vi "LFA_AcquireAltSPEMethod.vi"(8 "error in (no error)":errorcluster, 10 "Delete File?":bool, 11 "LightField Automation in":refnum<class "LightField Automation.lvclass">) -> (0 "error out":errorcluster, 2 "Data":T1(array[cluster]), 3 "LightField Automation out":refnum<class "LightField Automation.lvclass">)   [LabVIEW 2020, in "LightField Automation.lvclass"]
uses:
  LightField Automation.lvclass
  LightField Automation.lvclass/LightField Automation.ctl
  C:/Program Files/Princeton Instruments/LightField/AddInViews/PrincetonInstruments.LightFieldViewV3.dll
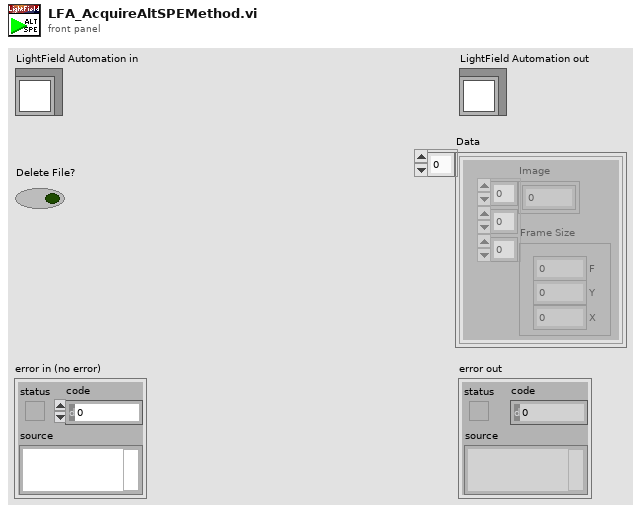
[diagram p1: front panel]
types:
  T1 = cluster{"Image":dbl[][][], "Frame Size":cluster{"F":i32, "Y":i32, "X":i32}}[]
  T2 = cluster{"ROI Height":i32[], "ROI Width":i32[], "ROI Stride":i32[], "ROI Size":i64[]}
  T3 = cluster{"Pixel Format":string, "Number of Frames":i32, "Frame Size":i32, "Frame Stride":i64}
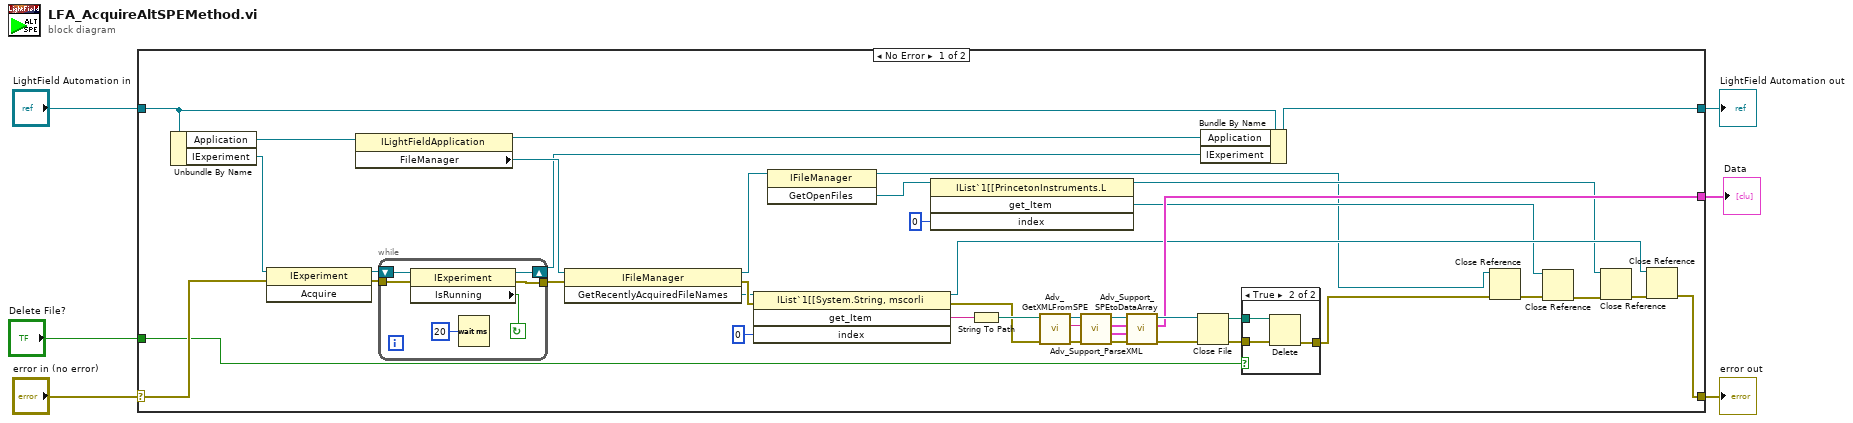
[diagram p0: block diagram]
diagram:
  n1 = case shown="No Error" "error in (no error)" {
    selector: "error in (no error)" -> [w48 w60]
    tunnel: [w20 w60] -> w5
    tunnel: [w26 w59] -> w3
    tunnel: "LightField Automation in" -> [w27 w59]
    tunnel: [w25 _] -> w2
    tunnel: "Delete File?" -> [w22 _]
    frame No Error {
      n2 = Unbundle By Name(w27) -> ("Application"=w44:refnum<k24>, "IExperiment"=w45:refnum<k24>)
      n3 = invoke class="IExperiment" method="Acquire"(reference=w45, error in=w48) -> (reference out=w46:refnum<k24>, error out=w47:errorcluster)  [unwired: 1 in, 1 out]
      n4 = property class="ILightFieldApplication"(reference=w44) -> (reference out=w16:refnum<k24>, "FileManager"=w43:refnum<k24>)  [unwired: 1 in, 1 out]
      n5 = while {
        tunnel: w47 -> [w56]
        tunnel: [w55] -> w42
        shift-right: [w53] -> w21
        shift-left: w46 -> [w54]
        stop <- w58 continue-if-true
        n6 = property class="IExperiment"(reference=w54, error in=w56) -> (reference out=w53:refnum<k24>, error out=w55:errorcluster, "IsRunning"=w58:bool)
        n7 = Wait (ms)(milliseconds to wait=u32 20) -> ()  [unwired: 1 out]
      }
      n8 = invoke class="IFileManager" method="GetRecentlyAcquiredFileNames"(reference=w43, error in=w42) -> (reference out=w15:refnum<k24>, error out=w41:errorcluster, "GetRecentlyAcquiredFileNames"=w19:refnum<k24>)  [unwired: 1 in]
      n9 = invoke class="IList`1[[System.String, mscorli" method="get_Item"(reference=w19, error in=w41, "index"=0) -> (reference out=w17:refnum<k24>, error out=w37:errorcluster, "get_Item"=w39:string)  [unwired: 1 in, 1 out]
      n10 = invoke class="IFileManager" method="GetOpenFiles"(reference=w15) -> (reference out=w7:refnum<k24>, "GetOpenFiles"=w14:refnum<k24>)  [unwired: 2 in, 1 out]
      n11 = invoke class="IList`1[[PrincetonInstruments.L" method="get_Item"(reference=w14, "index"=0) -> (reference out=w12:refnum<k24>, "get_Item"=w9:refnum<k24>)  [unwired: 2 in, 2 out]
      n12 = String To Path(string=w39) -> (path=w38:path)
      n13 = call "Adv_GetXMLFromSPE.vi"("error in (no error)"=w37, "Path In"=w38) -> ("error out"=w34:errorcluster, "XML"=w35:string, "SPE Refnum"=w36:refnum<file>)  [unwired: 7 in]
      n14 = call "Adv_Support_ParseXML.vi"("error in (no error)"=w34, "XML"=w35, "SPE Refnum"=w36) -> ("error out"=w30:errorcluster, "ROI Info"=w31:T2, "Frame Info"=w32:T3, "SPE Refnum"=w33:refnum<file>)  [unwired: 5 in]
      n15 = call "Adv_Support_SPEtoDataArray.vi"("error in (no error)"=w30, "ROI Info"=w31, "Frame Info"=w32, "SPE Refnum"=w33) -> ("error out"=w29:errorcluster, "Data"=w25:T1, "SPE Refnum 2"=w28:refnum<file>)  [unwired: 5 in]
      n16 = Close File(refnum=w28, error in=w29) -> (path=w23:path, error out=w24:errorcluster)
      n17 = Bundle By Name(cluster=w27, "Application"=w16, "IExperiment"=w21) -> (w26:refnum<class "LightField Automation.lvclass">)
      n18 = case shown="True" w22 {
        tunnel: w24 -> [w49 w52]
        tunnel: w23 -> [_ w51]
        tunnel: [w49 w50] -> w8
        frame False {
        }
        frame True {
          n19 = Delete(path (use dialog)=w51, error in=w52) -> (error out=w50:errorcluster)  [unwired: 3 in, 2 out]
        }
      }
      n20 = Close Reference(reference=w7, error in (no error)=w8) -> (error out=w11:errorcluster)
      n21 = Close Reference(reference=w9, error in (no error)=w11) -> (error out=w10:errorcluster)
      n22 = Close Reference(reference=w12, error in (no error)=w10) -> (error out=w18:errorcluster)
      n23 = Close Reference(reference=w17, error in (no error)=w18) -> (error out=w20:errorcluster)
    }
    frame Error {
    }
  }
  "error out" <- w5
  "LightField Automation out" <- w3
  "Data" <- w2
